vi "MoveIndicater.vi"(8 "error in (no error)":errorcluster, 10 "Indicator":i32, 11 "Panel_UI in":refnum<class "Panel_UI.lvclass">) -> (0 "error out":errorcluster, 3 "Panel_UI out":refnum<class "Panel_UI.lvclass">)   [LabVIEW 2015, in "Panel_UI.lvclass"]
uses:
  Panel_UI.lvclass
  Panel_UI.lvclass/Panel_UI.ctl
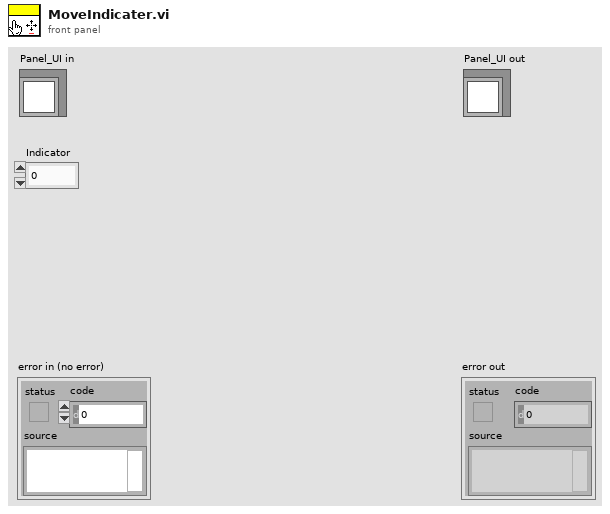
[diagram p1: front panel]
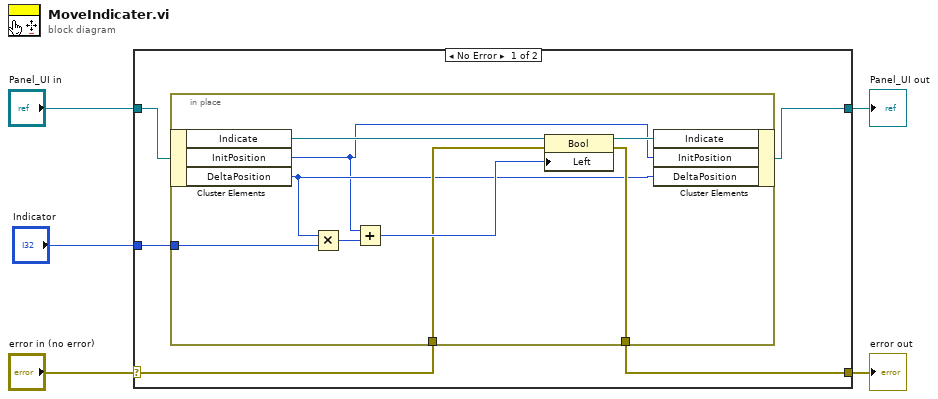
[diagram p0: block diagram]
diagram:
  n1 = case shown="No Error" "error in (no error)" {
    selector: "error in (no error)" -> [w10 w21]
    tunnel: [w7 w21] -> w4
    tunnel: [w6 w20] -> w2
    tunnel: "Panel_UI in" -> [w8 w20]
    tunnel: "Indicator" -> [w9 _]
    frame No Error {
      n2 = in-place {
        in-place-border: w10 -> [w13]
        in-place-border: w9 -> [w16]
        in-place-border: [w18] -> w7
        n3 = in-place-cluster #1(w8) -> ("Indicate"=w19:refnum<vi>, "InitPosition"=w11:i32, "DeltaPosition"=w12:i32)
        n4 = Multiply(x=w12, y=w16) -> (x*y=w15:i32)
        n5 = Add(x=w11, y=w15) -> (x+y=w14:i32)
        n6 = property class="Bool"(reference=w19, error in=w13, "Left"=w14) -> (reference out=w17:refnum<vi>, error out=w18:errorcluster)
        n7 = in-place-cluster #1("Indicate"=w17, "InitPosition"=w11, "DeltaPosition"=w12) -> (w6:refnum<class "Panel_UI.lvclass">)
      }
    }
    frame Error {
    }
  }
  "error out" <- w4
  "Panel_UI out" <- w2
